vi "Read existing settings.vi"(8 "error in (no error)":errorcluster, 10 "VI ref":refnum<vi>, 11 "refnum":T1) -> (0 "error out":errorcluster, 3 "refnum out":T1)   [LabVIEW 2025]
uses:
  <vilib>/Utility/config.llb/Config Data RefNum.ctl
  <userlib>/_OpenG.lib/variantconfig/variantconfig.llb/openg_variant_configuration_file.lvlib
  <vilib>/Utility/config.llb/NI_LVConfig.lvlib
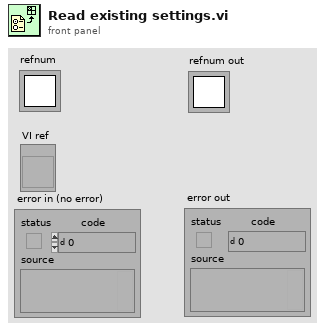
[diagram p1: front panel]
types:
  T1 = typedef "NI_LVConfig.lvlib/Config Data RefNum.ctl" = refnum<k1>
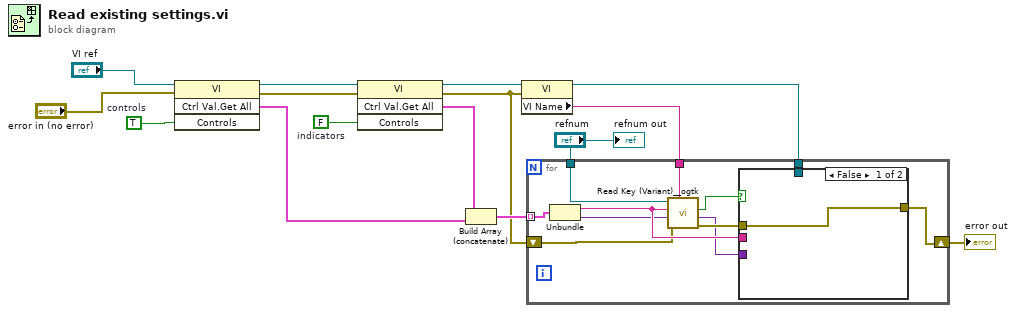
[diagram p0: block diagram]
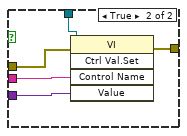
[diagram p2: hidden frame]
diagram:
  w13 = FALSE  # indicators
  w15 = TRUE  # controls
  n1 = invoke class="VI" method="Ctrl Val.Get All"(reference="VI ref", error in="error in (no error)", "Controls"=w15) -> (reference out=w14:refnum<vi>, error out=w9:errorcluster, "Get All Control Values Variant"=w11:cluster{"Name":string, "Variant Data":variant}[])  [unwired: 1 in, 1 out]
  n2 = invoke class="VI" method="Ctrl Val.Get All"(reference=w14, error in=w9, "Controls"=w13) -> (reference out=w10:refnum<vi>, error out=w4:errorcluster, "Get All Control Values Variant"=w12:cluster{"Name":string, "Variant Data":variant}[])  [unwired: 1 in, 1 out]
  n3 = Build Array (concatenate)(w12, w11) -> (w8:cluster{"Name":string, "Variant Data":variant}[])
  n4 = property class="VI"(reference=w10, error in=w4) -> (reference out=w1:refnum<vi>, "VI Name"=w7:string)  [unwired: 1 out]
  n5 = for {
    tunnel: w8 -> [w26] mode=indexing
    tunnel: w7 -> [w25]
    tunnel: "refnum" -> [w24]
    shift-right: [w22] -> w3
    shift-left: w4 -> [w18]
    tunnel: w1 -> [w23]
    n6 = Unbundle(w26) -> ("Name"=w20:string, "Variant Data"=w19:variant)
    n7 = call <userlib>:"Read Key (Variant)__ogtk.vi"("section"=w25, "error in (no error)"=w18, "type"=w19, "key (optional)"=w20, "refnum"=w24) -> ("error out"=w21:errorcluster, "key-value"=w17:variant, "found?"=w16:bool)  [unwired: 3 in, 1 out]
    n8 = case shown="False" w16 {
      tunnel: w23 -> [_ w32]
      tunnel: [w27 w31] -> w22
      tunnel: w21 -> [w27 w30]
      tunnel: w20 -> [_ w29]
      tunnel: w17 -> [_ w28]
      frame False {
      }
      frame True {
        n9 = invoke class="VI" method="Ctrl Val.Set"(reference=w32, error in=w30, "Control Name"=w29, "Value"=w28) -> (error out=w31:errorcluster)  [unwired: 1 in, 4 out]
      }
    }
  }
  "error out" <- w3
  "refnum out" <- "refnum"
